vi "2.vi"() -> ()   [LabVIEW 2023]
uses:
  1/TYPEDEF_COFFEE.ctl
  Control Timer.ctl
panel:
  out "error out":errorcluster
  out "Enum":T1
  in  "STOP":bool
  out "RELEASE ALL":bool
  out "MIXING":bool
  out "BOILING MILK":bool
  out "ADDING MILK":bool
  out "BOILING":bool
  out "ADDING COFFEE":bool
  out "ADDING WATER":bool
  in  "WHITE COFFEE":bool
  in  "CAPUCCINO":bool
  in  "ESPRESSO LONG":bool
  in  "ESPRESSO SHORT":bool
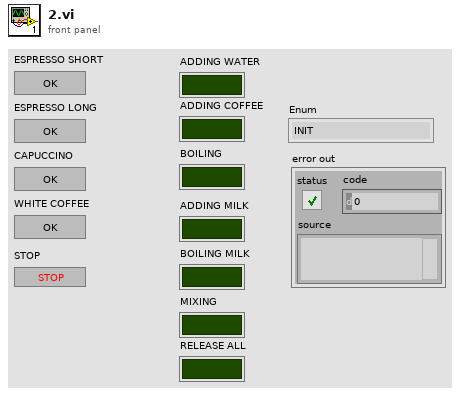
[diagram p1: front panel]
types:
  T1 = typedef "TYPEDEF_COFFEE.ctl" = enum16{"INIT", "WAIT", "SHUTDOWN", "ADDING WATER", "ADDING COFFEE", "BOILING", "ADDING MILK", "BOILING MILK", "MIXING", "RELEASE ALL"}
  T2 = typedef "Control Timer.ctl" = enum16{"Timecheck", "Reset"}
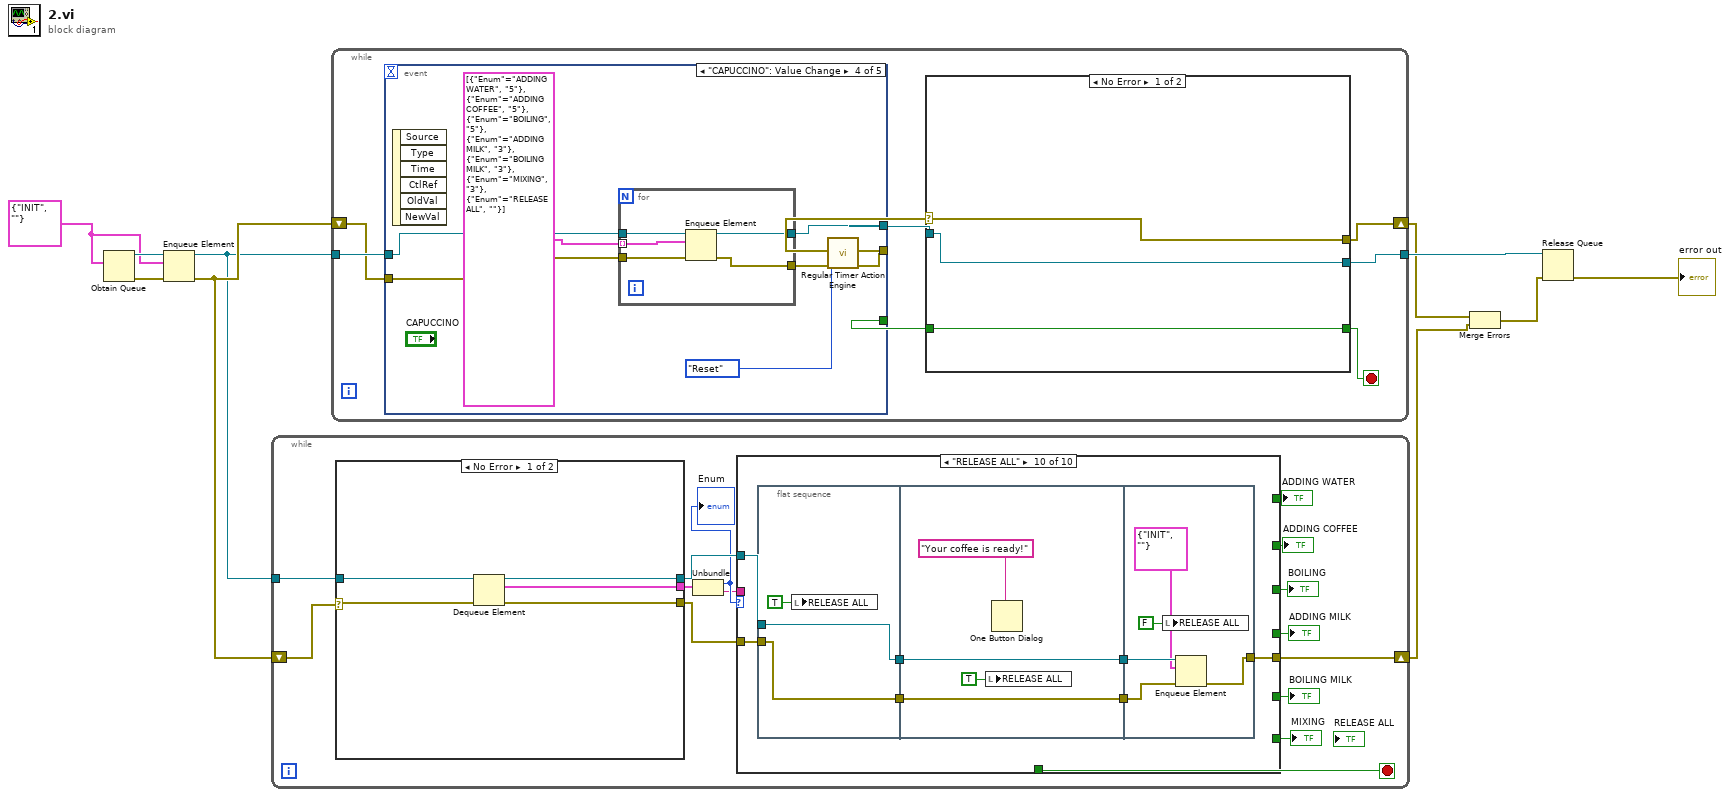
[diagram p0: block diagram]
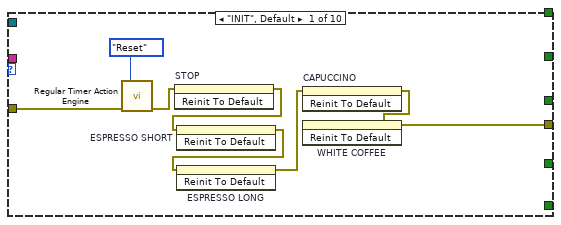
[diagram p2: hidden frame]
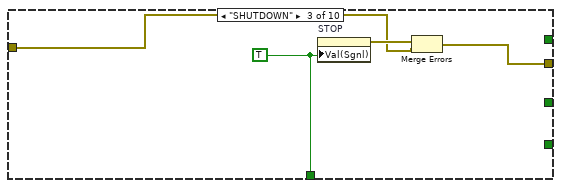
[diagram p4: hidden frame]
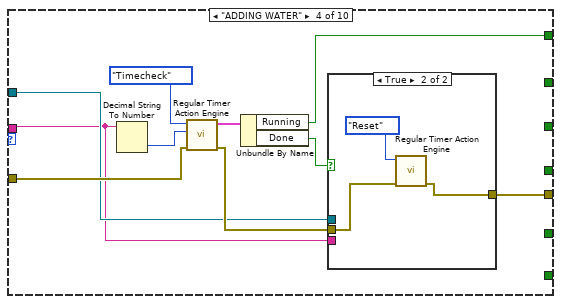
[diagram p5: hidden frame]
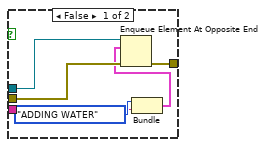
[diagram p6: hidden frame]
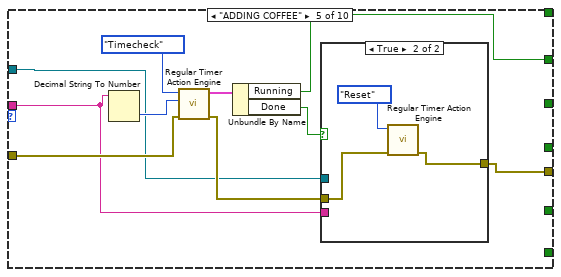
[diagram p7: hidden frame]
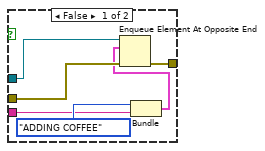
[diagram p8: hidden frame]
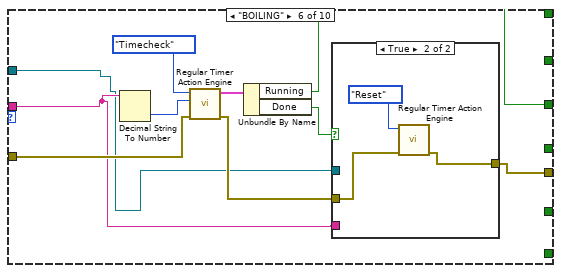
[diagram p9: hidden frame]
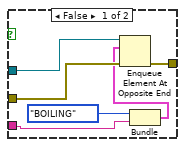
[diagram p10: hidden frame]
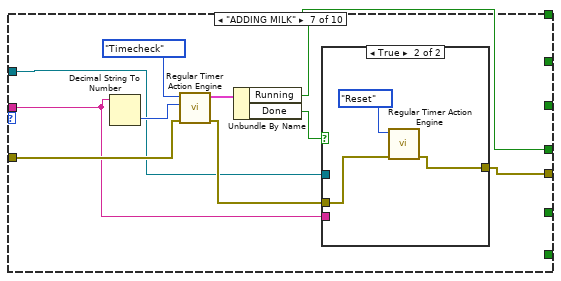
[diagram p11: hidden frame]
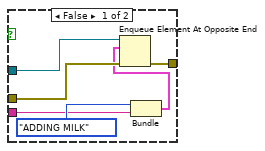
[diagram p12: hidden frame]
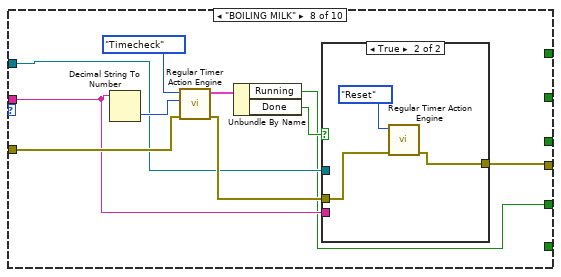
[diagram p13: hidden frame]
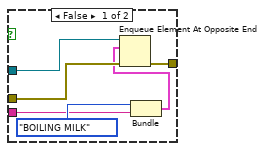
[diagram p14: hidden frame]
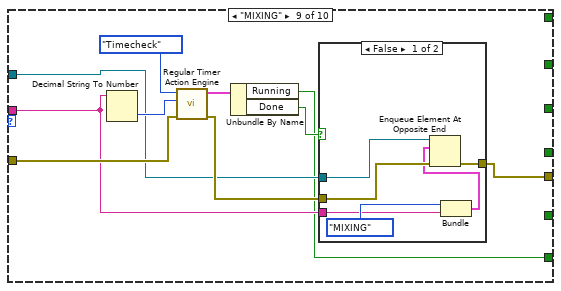
[diagram p15: hidden frame]
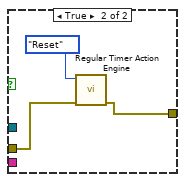
[diagram p16: hidden frame]
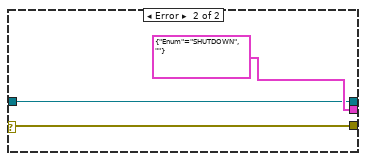
[diagram p17: hidden frame]
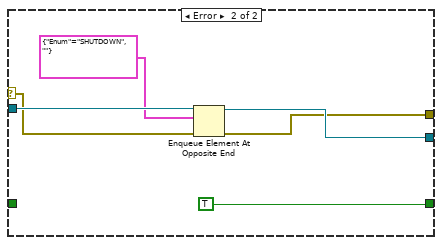
[diagram p18: hidden frame]
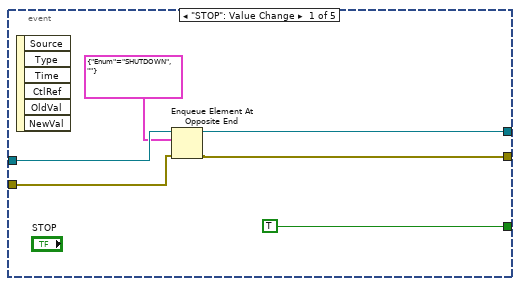
[diagram p19: hidden frame]
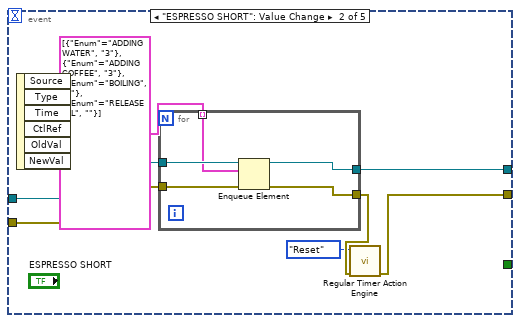
[diagram p20: hidden frame]
diagram:
  w8 = cluster{"Enum":T1, string} {"Enum"=enum."INIT", ""}
  n1 = Obtain Queue(element data type=w8) -> (queue out=w9:refnum<queue>, error out=w10:errorcluster)  [unwired: 4 in, 1 out]
  n2 = Enqueue Element(queue=w9, element=w8, error in (no error)=w10) -> (queue out=w6:refnum<queue>, error out=w7:errorcluster)  [unwired: 1 in, 1 out]
  n3 = while {
    shift-right: [w18] -> w4
    shift-left: w7 -> [w25]
    tunnel: w6 -> [w24]
    stop <- w17 stop-if-true
    n4 = case shown="No Error" w25 {
      selector: w25 -> [w176 w177]
      tunnel: w24 -> [w175 w178]
      tunnel: [w174 cluster{"Enum":T1, string} {"Enum"=enum."SHUTDOWN", ""} ("element")] -> w23
      tunnel: [w173 w178] -> w22
      tunnel: [w172 w177] -> w21
      frame No Error {
        n5 = Dequeue Element(queue=w175, error in (no error)=w176) -> (queue out=w173:refnum<queue>, element=w174:cluster{"Enum":T1, string}, error out=w172:errorcluster)  [unwired: 1 in, 1 out]
      }
      frame Error {
      }
    }
    n6 = Unbundle(w23) -> ("Enum"=w20:T1, w19:string)
    "Enum" <- w20
    n7 = case shown="\"RELEASE ALL\"" w20 {
      tunnel: w22 -> [_ _ _ w41 w61 w79 w99 w118 w137 w154]
      tunnel: w21 -> [w33 w34 w36 w45 w62 w81 w100 w119 w138 w159]
      tunnel: w19 -> [_ _ _ w39 w58 w80 w98 w117 w136 _]
      tunnel: [w26 w34 w35 w40 w59 w78 w96 w116 w135 w153] -> w18
      tunnel: [_ _ w38 _ _ _ _ _ _ _] -> w17
      tunnel: [_ _ _ w44 _ _ _ _ _ _] -> w16
      tunnel: [_ _ _ _ w60 _ _ _ _ _] -> w15
      tunnel: [_ _ _ _ _ w77 _ _ _ _] -> w14
      tunnel: [_ _ _ _ _ _ w97 _ _ _] -> w13
      tunnel: [_ _ _ _ _ _ _ w115 _ _] -> w12
      tunnel: [_ _ _ _ _ _ _ _ w134 _] -> w11
      frame "INIT", Default {
        n8 = call "Regular Timer Action Engine.vi"("Enum"=Control_Timer."Reset", "error in"=w33) -> ("error out"=w32:errorcluster)  [unwired: 7 in, 1 out]
        n9 = invoke on="STOP" class="Bool (strict)" method="Reinit To Default"(error in=w32) -> (error out=w31:errorcluster)  [unwired: 2 in, 2 out]
        n10 = invoke on="ESPRESSO SHORT" class="Bool" method="Reinit To Default"(error in=w31) -> (error out=w30:errorcluster)  [unwired: 2 in, 2 out]
        n11 = invoke on="ESPRESSO LONG" class="Bool" method="Reinit To Default"(error in=w30) -> (error out=w29:errorcluster)  [unwired: 2 in, 2 out]
        n12 = invoke on="CAPUCCINO" class="Bool" method="Reinit To Default"(error in=w29) -> (error out=w28:errorcluster)  [unwired: 2 in, 2 out]
        n13 = invoke on="WHITE COFFEE" class="Bool" method="Reinit To Default"(error in=w28) -> (error out=w26:errorcluster)  [unwired: 2 in, 2 out]
      }
      frame "WAIT" {
      }
      frame "SHUTDOWN" {
        w38 = TRUE
        n14 = property on="STOP" class="Bool (strict)"("Val(Sgnl)"=w38) -> (error out=w37:errorcluster)  [unwired: 2 in, 1 out]
        n15 = Merge Errors(w37, w36) -> (w35:errorcluster)
      }
      frame "ADDING WATER" {
        n16 = Decimal String To Number(string=w39) -> (number=w48:i32)  [unwired: 2 in, 1 out]
        n17 = call "Regular Timer Action Engine.vi"("Enum"=Control_Timer."Timecheck", "Time Target"=w48, "error in"=w45) -> ("Status"=w46:cluster{"Running":bool, "Done":bool}, "error out"=w42:errorcluster)  [unwired: 6 in]
        n18 = Unbundle By Name(w46) -> ("Running"=w44:bool, "Done"=w43:bool)
        n19 = case shown="True" w43 {
          tunnel: w42 -> [w53 w57]
          tunnel: w41 -> [w54 _]
          tunnel: [w52 w55] -> w40
          tunnel: w39 -> [w50 _]
          frame False {
            n20 = Bundle("Enum"=TYPEDEF_COFFEE."ADDING WATER", w50) -> (w49:cluster{"Enum":T1, string})  [unwired: 1 in]
            n21 = Enqueue Element At Opposite End(queue=w54, element=w49, error in (no error)=w53) -> (error out=w52:errorcluster)  [unwired: 1 in, 2 out]
          }
          frame True {
            n22 = call "Regular Timer Action Engine.vi"("Enum"=Control_Timer."Reset", "error in"=w57) -> ("error out"=w55:errorcluster)  [unwired: 7 in, 1 out]
          }
        }
      }
      frame "ADDING COFFEE" {
        n23 = Decimal String To Number(string=w58) -> (number=w67:i32)  [unwired: 2 in, 1 out]
        n24 = call "Regular Timer Action Engine.vi"("Enum"=Control_Timer."Timecheck", "Time Target"=w67, "error in"=w62) -> ("Status"=w65:cluster{"Running":bool, "Done":bool}, "error out"=w63:errorcluster)  [unwired: 6 in]
        n25 = Unbundle By Name(w65) -> ("Running"=w60:bool, "Done"=w64:bool)
        n26 = case shown="True" w64 {
          tunnel: w63 -> [w73 w76]
          tunnel: [w72 w74] -> w59
          tunnel: w61 -> [w71 _]
          tunnel: w58 -> [w69 _]
          frame False {
            n27 = Bundle("Enum"=TYPEDEF_COFFEE."ADDING COFFEE", w69) -> (w68:cluster{"Enum":T1, string})  [unwired: 1 in]
            n28 = Enqueue Element At Opposite End(queue=w71, element=w68, error in (no error)=w73) -> (error out=w72:errorcluster)  [unwired: 1 in, 2 out]
          }
          frame True {
            n29 = call "Regular Timer Action Engine.vi"("Enum"=Control_Timer."Reset", "error in"=w76) -> ("error out"=w74:errorcluster)  [unwired: 7 in, 1 out]
          }
        }
      }
      frame "BOILING" {
        n30 = Decimal String To Number(string=w80) -> (number=w86:i32)  [unwired: 2 in, 1 out]
        n31 = call "Regular Timer Action Engine.vi"("Enum"=Control_Timer."Timecheck", "Time Target"=w86, "error in"=w81) -> ("Status"=w84:cluster{"Running":bool, "Done":bool}, "error out"=w82:errorcluster)  [unwired: 6 in]
        n32 = Unbundle By Name(w84) -> ("Running"=w77:bool, "Done"=w83:bool)
        n33 = case shown="True" w83 {
          tunnel: w82 -> [w92 w95]
          tunnel: [w91 w93] -> w78
          tunnel: w80 -> [w89 _]
          tunnel: w79 -> [w88 _]
          frame False {
            n34 = Bundle("Enum"=TYPEDEF_COFFEE."BOILING", w89) -> (w87:cluster{"Enum":T1, string})  [unwired: 1 in]
            n35 = Enqueue Element At Opposite End(queue=w88, element=w87, error in (no error)=w92) -> (error out=w91:errorcluster)  [unwired: 1 in, 2 out]
          }
          frame True {
            n36 = call "Regular Timer Action Engine.vi"("Enum"=Control_Timer."Reset", "error in"=w95) -> ("error out"=w93:errorcluster)  [unwired: 7 in, 1 out]
          }
        }
      }
      frame "ADDING MILK" {
        n37 = Decimal String To Number(string=w98) -> (number=w105:i32)  [unwired: 2 in, 1 out]
        n38 = call "Regular Timer Action Engine.vi"("Enum"=Control_Timer."Timecheck", "Time Target"=w105, "error in"=w100) -> ("Status"=w103:cluster{"Running":bool, "Done":bool}, "error out"=w101:errorcluster)  [unwired: 6 in]
        n39 = Unbundle By Name(w103) -> ("Running"=w97:bool, "Done"=w102:bool)
        n40 = case shown="True" w102 {
          tunnel: w101 -> [w111 w114]
          tunnel: [w110 w112] -> w96
          tunnel: w99 -> [w108 _]
          tunnel: w98 -> [w107 _]
          frame False {
            n41 = Bundle("Enum"=TYPEDEF_COFFEE."ADDING MILK", w107) -> (w106:cluster{"Enum":T1, string})  [unwired: 1 in]
            n42 = Enqueue Element At Opposite End(queue=w108, element=w106, error in (no error)=w111) -> (error out=w110:errorcluster)  [unwired: 1 in, 2 out]
          }
          frame True {
            n43 = call "Regular Timer Action Engine.vi"("Enum"=Control_Timer."Reset", "error in"=w114) -> ("error out"=w112:errorcluster)  [unwired: 7 in, 1 out]
          }
        }
      }
      frame "BOILING MILK" {
        n44 = Decimal String To Number(string=w117) -> (number=w124:i32)  [unwired: 2 in, 1 out]
        n45 = call "Regular Timer Action Engine.vi"("Enum"=Control_Timer."Timecheck", "Time Target"=w124, "error in"=w119) -> ("Status"=w122:cluster{"Running":bool, "Done":bool}, "error out"=w120:errorcluster)  [unwired: 6 in]
        n46 = Unbundle By Name(w122) -> ("Running"=w115:bool, "Done"=w121:bool)
        n47 = case shown="True" w121 {
          tunnel: w120 -> [w130 w133]
          tunnel: [w129 w131] -> w116
          tunnel: w118 -> [w127 _]
          tunnel: w117 -> [w126 _]
          frame False {
            n48 = Bundle("Enum"=TYPEDEF_COFFEE."BOILING MILK", w126) -> (w125:cluster{"Enum":T1, string})  [unwired: 1 in]
            n49 = Enqueue Element At Opposite End(queue=w127, element=w125, error in (no error)=w130) -> (error out=w129:errorcluster)  [unwired: 1 in, 2 out]
          }
          frame True {
            n50 = call "Regular Timer Action Engine.vi"("Enum"=Control_Timer."Reset", "error in"=w133) -> ("error out"=w131:errorcluster)  [unwired: 7 in, 1 out]
          }
        }
      }
      frame "MIXING" {
        n51 = Decimal String To Number(string=w136) -> (number=w143:i32)  [unwired: 2 in, 1 out]
        n52 = call "Regular Timer Action Engine.vi"("Enum"=Control_Timer."Timecheck", "Time Target"=w143, "error in"=w138) -> ("Status"=w141:cluster{"Running":bool, "Done":bool}, "error out"=w139:errorcluster)  [unwired: 6 in]
        n53 = Unbundle By Name(w141) -> ("Running"=w134:bool, "Done"=w140:bool)
        n54 = case shown="False" w140 {
          tunnel: w139 -> [w149 w152]
          tunnel: [w148 w150] -> w135
          tunnel: w137 -> [w146 _]
          tunnel: w136 -> [w145 _]
          frame False {
            n55 = Bundle("Enum"=TYPEDEF_COFFEE."MIXING", w145) -> (w144:cluster{"Enum":T1, string})  [unwired: 1 in]
            n56 = Enqueue Element At Opposite End(queue=w146, element=w144, error in (no error)=w149) -> (error out=w148:errorcluster)  [unwired: 1 in, 2 out]
          }
          frame True {
            n57 = call "Regular Timer Action Engine.vi"("Enum"=Control_Timer."Reset", "error in"=w152) -> ("error out"=w150:errorcluster)  [unwired: 7 in, 1 out]
          }
        }
      }
      frame "RELEASE ALL" {
        n58 = flat-sequence {
          tunnel: w159 -> [w161]
          tunnel: [w161] -> w158
          tunnel: w154 -> [w160]
          tunnel: [w160] -> w155
          tunnel: w158 -> [w164]
          tunnel: [w164] -> w157
          tunnel: [w163] -> w156
          tunnel: w155 -> [w163]
          tunnel: w157 -> [w170]
          tunnel: w156 -> [w169]
          tunnel: [w168] -> w153
          frame #0 {
            n59 = local write "RELEASE ALL"(TRUE ("RELEASE ALL")) -> ()
          }
          frame #1 {
            n60 = local write "RELEASE ALL"(TRUE ("RELEASE ALL")) -> ()
            n61 = One Button Dialog(message="Your coffee is ready!") -> ()  [unwired: 1 in, 1 out]
          }
          frame #2 {
            n62 = local write "RELEASE ALL"(FALSE ("RELEASE ALL")) -> ()
            n63 = Enqueue Element(queue=w169, element=cluster{"Enum":T1, string} {"Enum"=enum."INIT", ""}, error in (no error)=w170) -> (error out=w168:errorcluster)  [unwired: 1 in, 2 out]
          }
        }
      }
    }
    "ADDING WATER" <- w16
    "ADDING COFFEE" <- w15
    "BOILING" <- w14
    "ADDING MILK" <- w13
    "BOILING MILK" <- w12
    "MIXING" <- w11
  }
  n64 = while {
    shift-right: [w180] -> w3
    shift-left: w7 -> [w186]
    tunnel: w6 -> [w187]
    tunnel: [w181] -> w5
    stop <- w183 stop-if-true
    n65 = event shown="[3] \"CAPUCCINO\": Value Change" {
      selector: _ -> [_ _ _ _ _]
      dyn-events: _ -> [_ _ _ _ _]
      timeout: _ -> [_ _ _ _ _]
      tunnel: w187 -> [w202 w208 w219 w230 w241]
      tunnel: w186 -> [w200 w209 w218 w231 w240]
      tunnel: [w199 w204 w221 w228 w243] -> w184
      tunnel: [w198 w206 w217 w232 w245] -> w182
      tunnel: [TRUE _ _ _ _] -> w185
      event "STOP": Value Change {
        n66 = event-data() -> ()  [unwired: 1 in, 6 out]
        n67 = Enqueue Element At Opposite End(queue=w202, element=cluster{"Enum":T1, string} {"Enum"=enum."SHUTDOWN", ""}, error in (no error)=w200) -> (queue out=w198:refnum<queue>, error out=w199:errorcluster)  [unwired: 1 in, 1 out]
      }
      event "ESPRESSO SHORT": Value Change {
        n68 = event-data() -> ()  [unwired: 1 in, 6 out]
        n69 = for {
          tunnel: w209 -> [w214]
          tunnel: w208 -> [w213]
          tunnel: cluster{"Enum":T1, string}[] [{"Enum"=enum."ADDING WATER", "3"}, {"Enum"=enum."ADDING COFFEE", "3"}, {"Enum"=enum."BOILING", "3"}, {"Enum"=enum."RELEASE ALL", ""}] -> [w212] mode=indexing
          tunnel: [w211] -> w205
          tunnel: [w210] -> w206
          n70 = Enqueue Element(queue=w213, element=w212, error in (no error)=w214) -> (queue out=w210:refnum<queue>, error out=w211:errorcluster)  [unwired: 1 in, 1 out]
        }
        n71 = call "Regular Timer Action Engine.vi"("Enum"=Control_Timer."Reset", "error in"=w205) -> ("error out"=w204:errorcluster)  [unwired: 7 in, 1 out]
      }
      event "ESPRESSO LONG": Value Change {
        n72 = event-data() -> ()  [unwired: 1 in, 6 out]
        n73 = for {
          tunnel: [w226] -> w220
          tunnel: w219 -> [w225]
          tunnel: w218 -> [w224]
          tunnel: [w223] -> w217
          tunnel: cluster{"Enum":T1, string}[] [{"Enum"=enum."ADDING WATER", "5"}, {"Enum"=enum."ADDING COFFEE", "5"}, {"Enum"=enum."BOILING", "5"}, {"Enum"=enum."RELEASE ALL", ""}] -> [w222] mode=indexing
          n74 = Enqueue Element(queue=w225, element=w222, error in (no error)=w224) -> (queue out=w223:refnum<queue>, error out=w226:errorcluster)  [unwired: 1 in, 1 out]
        }
        n75 = call "Regular Timer Action Engine.vi"("Enum"=Control_Timer."Reset", "error in"=w220) -> ("error out"=w221:errorcluster)  [unwired: 7 in, 1 out]
      }
      event "CAPUCCINO": Value Change {
        n76 = event-data() -> ()  [unwired: 1 in, 6 out]
        n77 = for {
          tunnel: [w238] -> w233
          tunnel: [w237] -> w232
          tunnel: w231 -> [w236]
          tunnel: w230 -> [w235]
          tunnel: cluster{"Enum":T1, string}[] [{"Enum"=enum."ADDING WATER", "5"}, {"Enum"=enum."ADDING COFFEE", "5"}, {"Enum"=enum."BOILING", "5"}, {"Enum"=enum."ADDING MILK", "3"}, {"Enum"=enum."BOILING MILK", "3"}, {"Enum"=enum."MIXING", "3"}, {"Enum"=enum."RELEASE ALL", ""}] -> [w234] mode=indexing
          n78 = Enqueue Element(queue=w235, element=w234, error in (no error)=w236) -> (queue out=w237:refnum<queue>, error out=w238:errorcluster)  [unwired: 1 in, 1 out]
        }
        n79 = call "Regular Timer Action Engine.vi"("Enum"=Control_Timer."Reset", "error in"=w233) -> ("error out"=w228:errorcluster)  [unwired: 7 in, 1 out]
      }
      event "WHITE COFFEE": Value Change {
        n80 = event-data() -> ()  [unwired: 1 in, 6 out]
        n81 = for {
          tunnel: [w250] -> w245
          tunnel: [w249] -> w244
          tunnel: w241 -> [w248]
          tunnel: w240 -> [w247]
          tunnel: cluster{"Enum":T1, string}[] [{"Enum"=enum."ADDING MILK", "5"}, {"Enum"=enum."ADDING COFFEE", "2"}, {"Enum"=enum."BOILING MILK", "5"}, {"Enum"=enum."RELEASE ALL", ""}] -> [w246] mode=indexing
          n82 = Enqueue Element(queue=w248, element=w246, error in (no error)=w247) -> (queue out=w250:refnum<queue>, error out=w249:errorcluster)  [unwired: 1 in, 1 out]
        }
        n83 = call "Regular Timer Action Engine.vi"("Enum"=Control_Timer."Reset", "error in"=w244) -> ("error out"=w243:errorcluster)  [unwired: 7 in, 1 out]
      }
    }
    n84 = case shown="No Error" w184 {
      selector: w184 -> [w188 w193]
      tunnel: w185 -> [w190 _]
      tunnel: [w190 TRUE] -> w183
      tunnel: w182 -> [w189 w196]
      tunnel: [w189 w195] -> w181
      tunnel: [w188 w194] -> w180
      frame No Error {
      }
      frame Error {
        n85 = Enqueue Element At Opposite End(queue=w196, element=cluster{"Enum":T1, string} {"Enum"=enum."SHUTDOWN", ""}, error in (no error)=w193) -> (queue out=w195:refnum<queue>, error out=w194:errorcluster)  [unwired: 1 in, 1 out]
      }
    }
  }
  n86 = Merge Errors(w3, w4) -> (w2:errorcluster)
  n87 = Release Queue(queue=w5, error in (no error)=w2) -> (error out=→"error out":errorcluster)  [unwired: 1 in, 2 out]
